vi "S2C_UpdateGlobals.vi"(8 "Error In":errorcluster, 9 "Values":string[](array[string]), 10 "Keys":string[](array[string]), 11 "Section":string) -> (0 "Error Out":errorcluster)   [LabVIEW 2015]
doc: "Loads setting file values into their respective globals."
uses:
  Globals/S2C_Globals.vi
  Globals/S2C_GlobalMenus.vi
  Core/Process/Fornax/VIs/S2C_FORNAX_Proc_Globals.vi
  Core/Process/PCIe7841/VIs/S2C_PCIe7841_Proc_Globals.vi
  XML/S2C_XML_Globals.vi
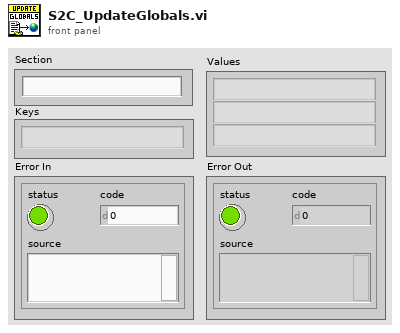
[diagram p1: front panel]
types:
  T1 = cluster{"EventName":string, "ProcessName":string, "ProductLine":string, "EventStatus":string, "EventStart":string, "EventStop":string, "Station":string, "OperatorName":string, "Location":string}
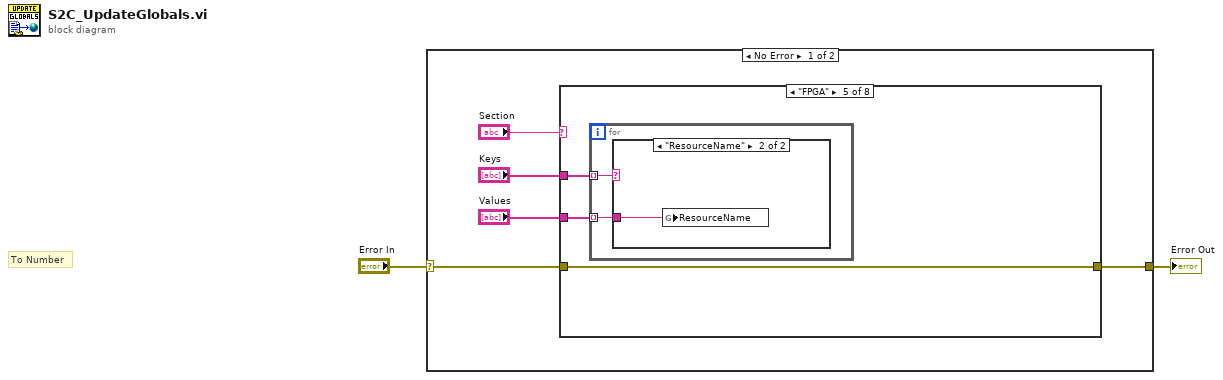
[diagram p0: block diagram]
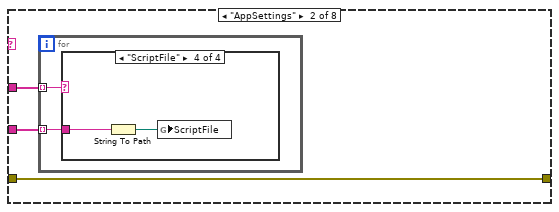
[diagram p3: hidden frame]
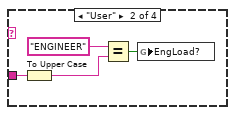
[diagram p5: hidden frame]
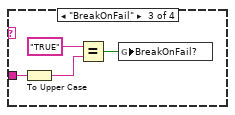
[diagram p6: hidden frame]
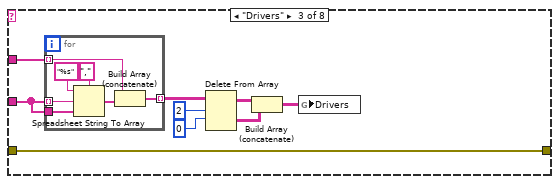
[diagram p7: hidden frame]
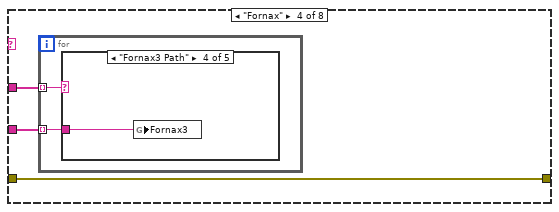
[diagram p8: hidden frame]
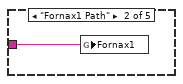
[diagram p10: hidden frame]
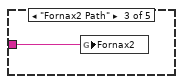
[diagram p11: hidden frame]
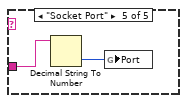
[diagram p12: hidden frame]
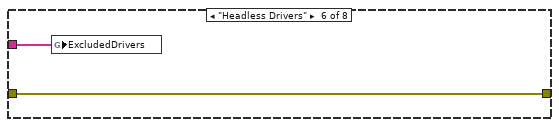
[diagram p14: hidden frame]
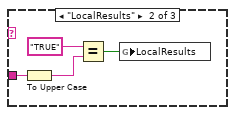
[diagram p16: hidden frame]
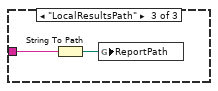
[diagram p17: hidden frame]
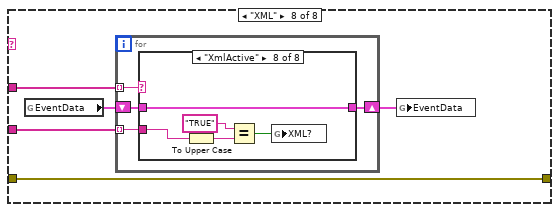
[diagram p18: hidden frame]
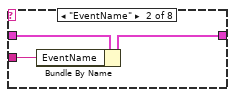
[diagram p20: hidden frame]
diagram:
  # "To Number"
  n1 = case shown="No Error" "Error In" {
    selector: "Error In" -> [w7 w102]
    tunnel: [w3 w102] -> w1
    frame No Error {
      n2 = case shown="\"FPGA\"" "Section" {
        tunnel: "Values" -> [_ w10 w31 w41 w51 w56 w59 w72]
        tunnel: w7 -> [w8 w9 w32 w40 w50 w57 w58 w71]
        tunnel: [w8 w9 w32 w40 w50 w57 w58 w71] -> w3
        tunnel: "Keys" -> [_ w11 w30 w42 w52 _ w60 w73]
        frame "Other", Default {
        }
        frame "AppSettings" {
          n3 = for {
            tunnel: w11 -> [w13] mode=indexing
            tunnel: w10 -> [w12] mode=indexing
            n4 = case shown="\"ScriptFile\"" w13 {
              tunnel: w12 -> [_ w17 w21 w23]
              frame "Unknown", Default {
              }
              frame "User" {
                n5 = To Upper Case(1:w17) -> (0:w16:string)
                n6 = Equal?(x="ENGINEER", y=w16) -> (x = y?=w14:bool)
                n7 = global write "S2C_Globals.vi" "EngLoad?"(w14) -> ()
              }
              frame "BreakOnFail" {
                n8 = To Upper Case(1:w21) -> (0:w20:string)
                n9 = Equal?(x="TRUE", y=w20) -> (x = y?=w18:bool)
                n10 = global write "S2C_Globals.vi" "BreakOnFail?"(w18) -> ()
              }
              frame "ScriptFile" {
                n11 = String To Path(string=w23) -> (path=w22:path)
                n12 = global write "S2C_Globals.vi" "ScriptFile"(w22) -> ()
              }
            }
          }
        }
        frame "Drivers" {
          n13 = for {
            tunnel: w31 -> [w39] mode=indexing
            tunnel: w31 -> [w38]
            tunnel: w30 -> [w34] mode=indexing
            tunnel: [w33] -> w29 mode=indexing
            n14 = Spreadsheet String To Array(delimiter (Tab)=",", format string="%s", spreadsheet string=w39, array type (2D Dbl)=w38) -> (array=w35:string[])
            n15 = Build Array (concatenate)(w34, w35) -> (w33:string[])
          }
          n16 = Delete From Array(array=w29, length=2, index (row)=0) -> (deleted portion=w26:string[][], array with subset deleted=w27:string[][])  [unwired: 1 in]
          n17 = Build Array (concatenate)(w27, w26) -> (w25:string[][])
          n18 = global write "S2C_GlobalMenus.vi" "Drivers"(w25) -> ()
        }
        frame "Fornax" {
          n19 = for {
            tunnel: w42 -> [w44] mode=indexing
            tunnel: w41 -> [w43] mode=indexing
            n20 = case shown="\"Fornax3 Path\"" w44 {
              tunnel: w43 -> [_ w45 w46 w47 w49]
              frame "Unknown", Default {
              }
              frame "Fornax1 Path" {
                n21 = global write "S2C_FORNAX_Proc_Globals.vi" "Fornax1"(w45) -> ()
              }
              frame "Fornax2 Path" {
                n22 = global write "S2C_FORNAX_Proc_Globals.vi" "Fornax2"(w46) -> ()
              }
              frame "Fornax3 Path" {
                n23 = global write "S2C_FORNAX_Proc_Globals.vi" "Fornax3"(w47) -> ()
              }
              frame "Socket Port" {
                n24 = Decimal String To Number(string=w49) -> (number=w48:i32)  [unwired: 2 in, 1 out]
                n25 = global write "S2C_FORNAX_Proc_Globals.vi" "Port"(w48) -> ()
              }
            }
          }
        }
        frame "FPGA" {
          n26 = for {
            tunnel: w52 -> [w54] mode=indexing
            tunnel: w51 -> [w53] mode=indexing
            n27 = case shown="\"ResourceName\"" w54 {
              tunnel: w53 -> [_ w55]
              frame "Unknown", Default {
              }
              frame "ResourceName" {
                n28 = global write "S2C_PCIe7841_Proc_Globals.vi" "ResourceName"(w55) -> ()
              }
            }
          }
        }
        frame "Headless Drivers" {
          n29 = global write "S2C_GlobalMenus.vi" "ExcludedDrivers"(w56) -> ()
        }
        frame "Output" {
          n30 = for {
            tunnel: w60 -> [w62] mode=indexing
            tunnel: w59 -> [w61] mode=indexing
            n31 = case shown="\"Unknown\", Default" w62 {
              tunnel: w61 -> [_ w66 w68]
              frame "Unknown", Default {
              }
              frame "LocalResults" {
                n32 = To Upper Case(1:w66) -> (0:w65:string)
                n33 = Equal?(x="TRUE", y=w65) -> (x = y?=w63:bool)
                n34 = global write "S2C_Globals.vi" "LocalResults"(w63) -> ()
              }
              frame "LocalResultsPath" {
                n35 = String To Path(string=w68) -> (path=w67:path)
                n36 = global write "S2C_Globals.vi" "ReportPath"(w67) -> ()
              }
            }
          }
        }
        frame "XML" {
          n37 = global read "S2C_XML_Globals.vi" "EventData"() -> (w70:T1)
          n38 = for {
            tunnel: w73 -> [w77] mode=indexing
            tunnel: w72 -> [w76] mode=indexing
            shift-right: [w74] -> w69
            shift-left: w70 -> [w75]
            n39 = case shown="\"XmlActive\"" w77 {
              tunnel: w76 -> [_ w80 w83 w86 w89 w92 w96 w101]
              tunnel: w75 -> [w78 w81 w84 w87 w90 w93 w95 w97]
              tunnel: [w78 w79 w82 w85 w88 w91 w95 w97] -> w74
              frame "Unknown", Default {
              }
              frame "EventName" {
                n40 = Bundle By Name(cluster=w81, "EventName"=w80) -> (w79:T1)
              }
              frame "ProcessName" {
                n41 = Bundle By Name(cluster=w84, "ProcessName"=w83) -> (w82:T1)
              }
              frame "ProductLine" {
                n42 = Bundle By Name(cluster=w87, "ProductLine"=w86) -> (w85:T1)
              }
              frame "Station" {
                n43 = Bundle By Name(cluster=w90, "Station"=w89) -> (w88:T1)
              }
              frame "OperatorName" {
                n44 = Bundle By Name(cluster=w93, "OperatorName"=w92) -> (w91:T1)
              }
              frame "XmlPath" {
                n45 = String To Path(string=w96) -> (path=w94:path)
                n46 = global write "S2C_XML_Globals.vi" "XML_Output"(w94) -> ()
              }
              frame "XmlActive" {
                n47 = To Upper Case(1:w101) -> (0:w100:string)
                n48 = Equal?(x="TRUE", y=w100) -> (x = y?=w98:bool)
                n49 = global write "S2C_XML_Globals.vi" "XML?"(w98) -> ()
              }
            }
          }
          n50 = global write "S2C_XML_Globals.vi" "EventData"(w69) -> ()
        }
      }
    }
    frame Error {
    }
  }
  "Error Out" <- w1
